vi "I-V扫描.vi"(8 "错误输入":errorcluster, 10 "参数":T1, 11 "VISA资源名称":refnum<visa-resource-name>) -> (0 "错误输出":errorcluster, 3 "VISA资源名称输出":refnum<visa-resource-name>)   [LabVIEW 2019]
uses:
  lib/Global variable.vi
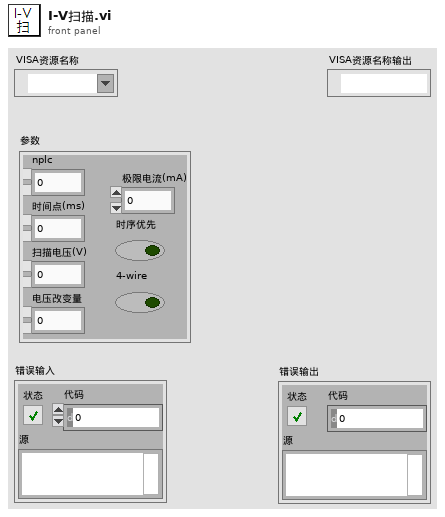
[diagram p1: front panel]
types:
  T1 = cluster{"nplc":dbl, "时序优先":bool, "时间点(ms)":dbl, "电压改变量":dbl, "极限电流(mA)":dbl, "扫描电压(V)":dbl, "4-wire ":bool}
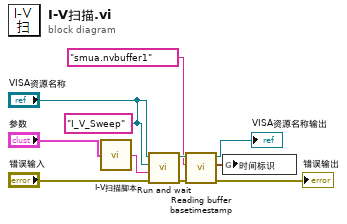
[diagram p0: block diagram]
diagram:
  w1 = "I_V_Sweep" ("Script Name")
  n1 = call "I-V扫描脚本.vi"("参数"="参数") -> ("Script"=w8:string)
  n2 = call "Run and wait.vi"("错误输入"="错误输入", "Script"=w8, "Script Name"="VISA资源名称", "VISA资源名称"="VISA资源名称") -> ("错误输出"=w4:errorcluster, "VISA资源名称输出"=w5:refnum<visa-resource-name>)  [unwired: 6 in]
  n3 = call "Reading buffer basetimestamp.vi"("错误输入"=w4, "缓冲区名称"="smua.nvbuffer1", "VISA资源名称"=w5) -> ("错误输出"=→"错误输出":errorcluster, "时间标识"=w2:timestamp, "VISA资源名称输出"=→"VISA资源名称输出":refnum<visa-resource-name>)  [unwired: 6 in]
  n4 = global write "Global variable.vi" "时间标识"(w2) -> ()
